vi "TIFF camera test 2.vi"(8 "Gain":i32=100 min=100 max=2000 step=1, 9 "Exposure time (ms)":dbl=100.0 min=1.0 max=10000.0 step=1.0) -> (2 "Image out":T1(plugin-control))   [LabVIEW 2017]
uses:
  libtiff/ctiff.llb/__CTIFFNewFileAndStyleUINT16.vi
  libtiff/ctiff.llb/__CTIFFAddNewPageUINT16.vi
panel:
  out "Capturing":bool
  in  "TIF file path":path=path "C:/Users/Chip Scope/Desktop/test.tif"
  in  "stop":bool
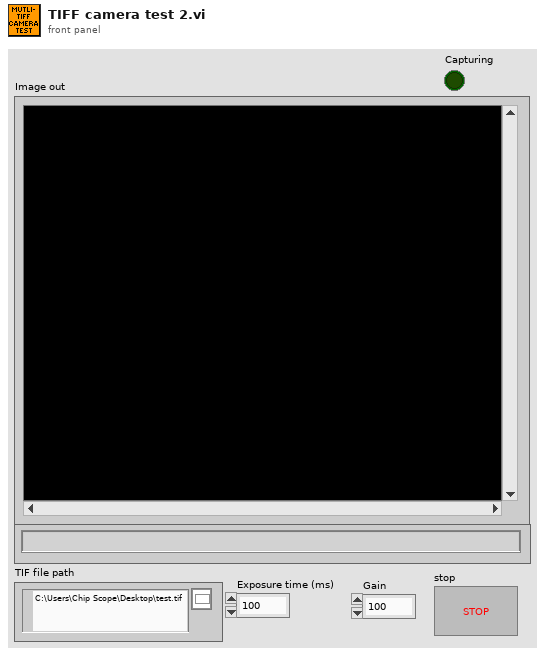
[diagram p1: front panel]
types:
  T1 = typedef "IMAQ Image.ctl" = refnum<image>
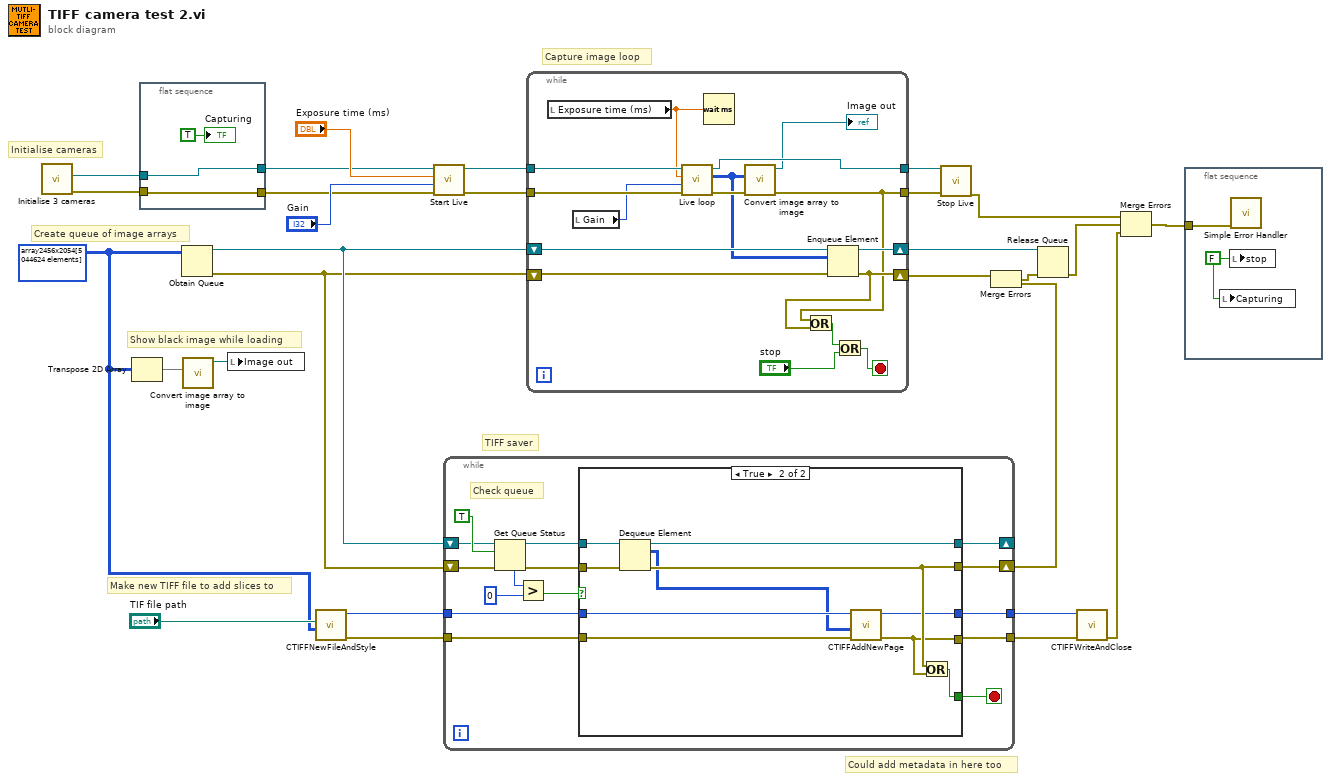
[diagram p0: block diagram]
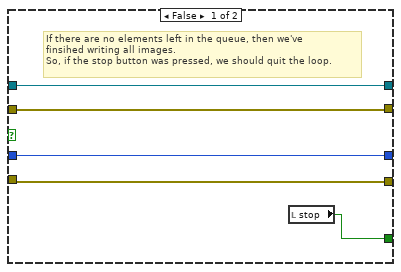
[diagram p2: hidden frame]
diagram:
  w7 = u16[][] array2456x2054[5044624 elements] ("Image Array")
  # "Show black image while loading"
  # "Could add metadata in here too"
  # "Make new TIFF file to add slices to"
  # "Initialise cameras"
  # "Create queue of image arrays"
  # "TIFF saver"
  # "Capture image loop"
  n1 = call "Initialise 3 cameras.vi"() -> ("Error Out"=w4:errorcluster, "Green camera ref"=w1:refnum<k24>)  [unwired: 8 in, 2 out]
  n2 = Transpose 2D Array(2D array=w7) -> (transposed array=w6:u16[][])
  n3 = flat-sequence {
    tunnel: w4 -> [w31]
    tunnel: [w31] -> w3
    tunnel: w1 -> [w30]
    tunnel: [w30] -> w2
    frame #0 {
      "Capturing" <- TRUE ("Capturing")
    }
  }
  n4 = Obtain Queue(element data type=w7) -> (queue out=w20:refnum<queue>, error out=w19:errorcluster)  [unwired: 4 in, 1 out]
  n5 = call "Convert image array to image.vi"("Array"=w6) -> ("Image Out"=w5:T1)  [unwired: 8 in, 1 out]
  n6 = local write "Image out"(w5) -> ()
  n7 = call-poly "CTIFFNewFileAndStyle.vi"("image"=w7, "output_file"="TIF file path") -> ("error"=w11:errorcluster, "CTIFF"=w12:i64)  [unwired: 8 in]
  n8 = call "Start Live.vi"("Error In"=w3, "Gain in"="Gain", "Exposure time (ms)"="Exposure time (ms)", "Camera reference in"=w2) -> ("Error Out"=w17:errorcluster, "Camera reference out"=w14:refnum<k24>)  [unwired: 5 in]
  n9 = while {
    shift-right: [w46] -> _
    shift-left: w20 -> [w36]
    shift-right: [w44] -> w18
    shift-left: w19 -> [w39]
    tunnel: w12 -> [w35]
    tunnel: w11 -> [w34]
    tunnel: [w33] -> w10
    tunnel: [w32] -> w9
    stop <- w45 stop-if-true
    # "Check queue"
    n10 = Get Queue Status(queue=w36, return elements? (F)=TRUE, error in (no error)=w39) -> (queue out=w37:refnum<queue>, error out=w38:errorcluster, # elements in queue=w42:i32)  [unwired: 5 out]
    n11 = Greater?(x=w42, y=0) -> (0:w40:bool)
    n12 = case shown="True" w40 {
      tunnel: w37 -> [w51 w61]
      tunnel: w38 -> [w50 w60]
      tunnel: [w51 w59] -> w46
      tunnel: [w47 w58] -> w45
      tunnel: [w50 w57] -> w44
      tunnel: w35 -> [w49 w56]
      tunnel: w34 -> [w48 w55]
      tunnel: [w49 w54] -> w33
      tunnel: [w48 w53] -> w32
      frame False {
        # "If there are no elements left in the queue, then we've \nfinsihed writing all images. \nSo, if the stop button was pressed, we should quit the loop."
        n13 = local read "stop"() -> (w47:bool)
      }
      frame True {
        n14 = Dequeue Element(queue=w61, error in (no error)=w60) -> (queue out=w59:refnum<queue>, element=w52:u16[][], error out=w57:errorcluster)  [unwired: 1 in, 1 out]
        n15 = call-poly "CTIFFAddNewPage.vi"("error"=w55, "image"=w52, "CTIFF"=w56) -> ("error"=w53:errorcluster, "CTIFF"=w54:i64)  [unwired: 7 in]
        n16 = Or(x=w57, y=w53) -> (x .or. y?=w58:bool)
      }
    }
  }
  n17 = while {
    tunnel: [w64] -> w28
    tunnel: [w77] -> w27
    tunnel: w14 -> [w76]
    tunnel: w17 -> [w75]
    shift-right: [w68] -> w26
    shift-left: w20 -> [w70]
    shift-right: [w67] -> w24
    shift-left: w19 -> [w69]
    stop <- w71 stop-if-true
    n18 = local read "Exposure time (ms)"() -> (w62:dbl)
    n19 = local read "Gain"() -> (w74:i32)
    n20 = call "Live loop.vi"("Error In"=w75, "Gain"=w74, "Exposure time (ms)"=w62, "Camera reference in"=w76) -> ("Error Out"=w65:errorcluster, "Image Array"=w63:u16[][], "Camera reference out"=w77:refnum<k24>)  [unwired: 4 in]
    n21 = Wait (ms)(milliseconds to wait=w62) -> ()  [unwired: 1 out]
    n22 = call "Convert image array to image.vi"("Error In"=w65, "Array"=w63) -> ("error out"=w64:errorcluster, "Image Out"=→"Image out":T1)  [unwired: 7 in]
    n23 = Enqueue Element(queue=w70, element=w63, error in (no error)=w69) -> (queue out=w68:refnum<queue>, error out=w67:errorcluster)  [unwired: 1 in, 1 out]
    n24 = Or(x=w64, y=w67) -> (x .or. y?=w73:bool)
    n25 = Or(x=w73, y="stop") -> (x .or. y?=w71:bool)
  }
  n26 = call "Stop Live.vi"("Camera reference in"=w27, "Error In"=w28) -> ("Error Out"=w23:errorcluster)  [unwired: 16 in, 1 out]
  n27 = Merge Errors(w24, w18) -> (w25:errorcluster)
  n28 = Release Queue(queue=w26, error in (no error)=w25) -> (error out=w22:errorcluster)  [unwired: 1 in, 2 out]
  n29 = call "CTIFFWriteAndClose.vi"("error"=w9, "CTIFF"=w10) -> ("error"=w8:errorcluster)  [unwired: 9 in]
  n30 = Merge Errors(w23, w22, w8) -> (w21:errorcluster)
  n31 = flat-sequence {
    tunnel: w21 -> [w79]
    frame #0 {
      w78 = FALSE ("stop")
      n32 = local write "Capturing"(w78) -> ()
      n33 = local write "stop"(w78) -> ()
      n34 = call <vilib>:"Simple Error Handler.vi"("error in (no error)"=w79) -> ()  [unwired: 4 in, 5 out]
    }
  }
